vi "backup_stepper_Control.vi"   [LabVIEW 2015]
uses:
  <vilib>/eio/EIOMethodNode/EIOMethodNode.xnode
  <vilib>/rvi/eio/common/nirviEmuTemplateMethod_errors.vi
  <vilib>/eio/EIOPropertyNode/EIOPropertyNode.xnode
  <vilib>/eio/EIONode/EIONode.xnode
  Controls/Stepper SM Enumerator.ctl
  <vilib>/rvi/eio/common/nirviEmuTemplatePropertyGet_errors.vi
  <vilib>/rvi/eio/common/nirviEmuTemplatePropertyGet_noerrors.vi
  <vilib>/rvi/eio/common/nirviEmuTemplatePropertySet_errors.vi
  <vilib>/rvi/eio/common/nirviEmuTemplatePropertySet_noerrors.vi
types:
  T1 = typedef "Stepper SM Enumerator.ctl" = enum16{"Running", "Backing up", "Idle", "Home", "Lim"}
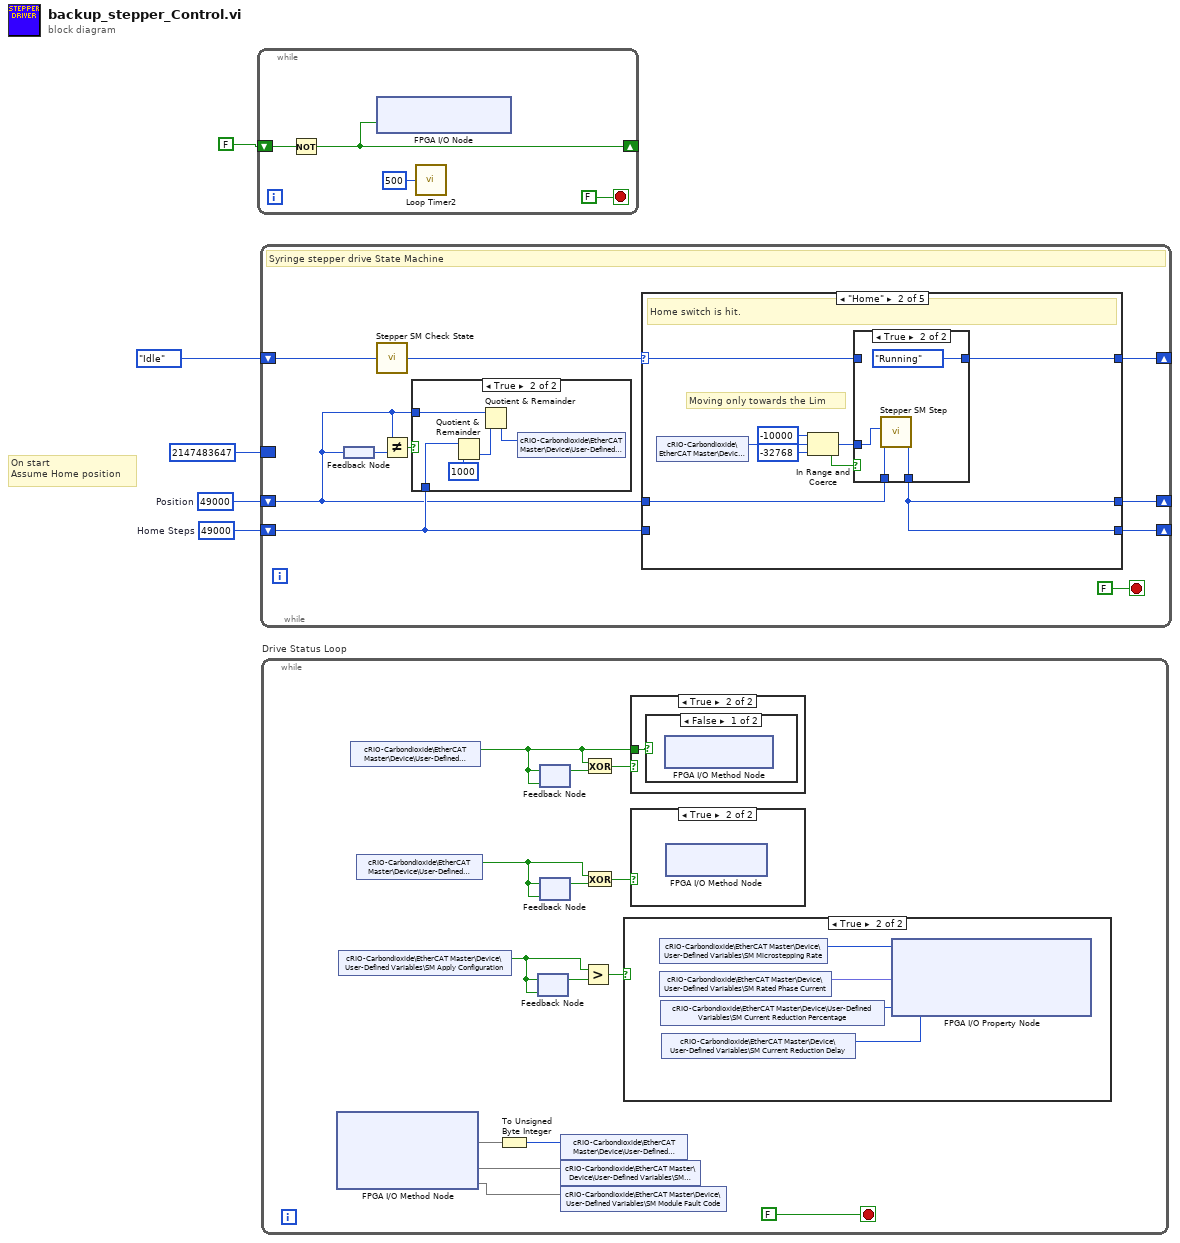
[diagram p0: block diagram]
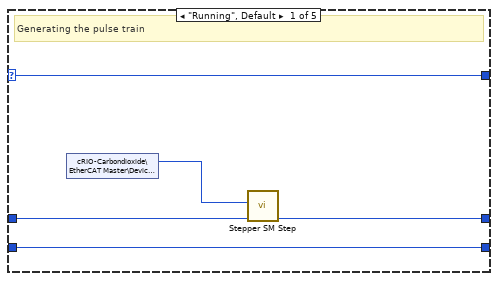
[diagram p3: hidden frame]
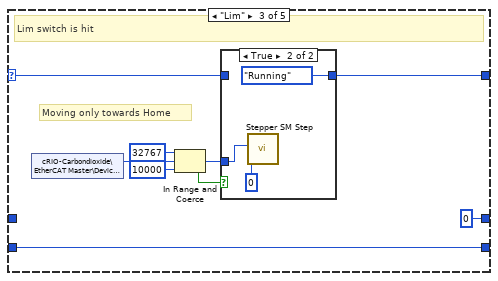
[diagram p5: hidden frame]
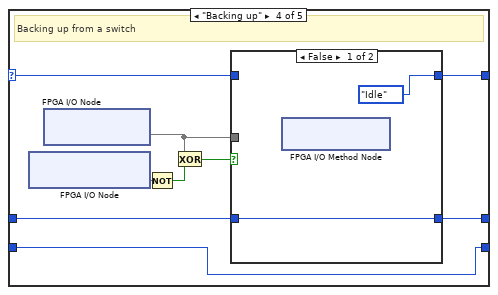
[diagram p7: hidden frame]
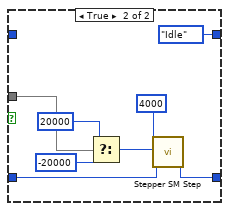
[diagram p8: hidden frame]
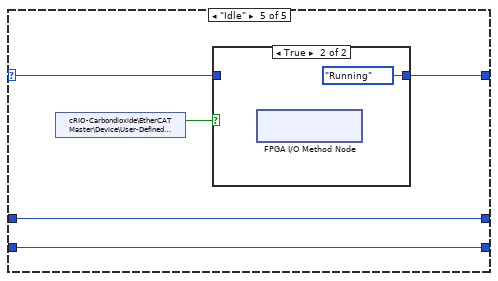
[diagram p9: hidden frame]
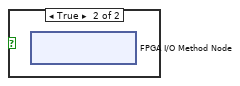
[diagram p14: hidden frame]
diagram:
  w1 = 49000  # Home Steps
  w3 = 49000  # Position
  # "On start\nAssume Home position"
  n1 = while {
    shift-right: [w7] -> _
    shift-left: FALSE ("Stepper/User LED") -> [w8]
    stop <- FALSE stop-if-true
    n2 = Not(x=w8) -> (.not. x?=w7:bool)
    n3 = xnode "FPGA I/O Node"("Stepper/User LED"=w7) -> ()  [unwired: 1 in, 1 out]
    n4 = call "Loop Timer2"("Count(mSec)"=u32 500) -> ()  [unwired: 1 out]
  }
  n5 = while {
    shift-right: [w18] -> _
    shift-left: Stepper_SM_Enumerator."Idle" -> [w17]
    shift-right: [w15] -> _
    shift-left: w3 -> [w10]
    border: 2147483647 -> [_]
    shift-right: [w13] -> _
    shift-left: w1 -> [w11]
    stop <- FALSE stop-if-true
    # "Syringe stepper drive State Machine"
    n6 = feedback-in #1(w10) -> ()
    n7 = feedback #1() -> (w12:i32)
    n8 = call "Stepper SM Check State.vi"("State in"=w17) -> ("State out"=w16:T1)
    n9 = Not Equal?(x=w10, y=w12) -> (x != y?=w14:bool)
    n10 = case shown="True" w14 {
      tunnel: w10 -> [_ w21]
      tunnel: w11 -> [_ w20]
      frame False {
      }
      frame True {
        n11 = Quotient & Remainder(x=w20, y=1000) -> (floor(x/y)=w23:i32)  [unwired: 1 out]
        n12 = Quotient & Remainder(x=w21, y=w23) -> (floor(x/y)=w22:i32)  [unwired: 1 out]
        n13 = shared-variable "cRIO-Carbondioxide\\EtherCAT Master\\Device\\User-Defined Variables\\SM Position"(w22) -> ()  [unwired: 1 in, 1 out]
      }
    }
    n14 = case shown="\"Home\"" w16 {
      selector: w16 -> [w29 w32 w48 w63 w80]
      tunnel: [w29 w33 w47 w61 w79] -> w18
      tunnel: w10 -> [w27 w31 _ w60 w78]
      tunnel: [w26 w30 0 ("Position") w59 w78] -> w15
      tunnel: [w25 w30 w46 w58 w77] -> w13
      tunnel: w11 -> [w25 _ w46 w58 w77]
      frame "Running", Default {
        # "Generating the pulse train"
        n15 = shared-variable "cRIO-Carbondioxide\\EtherCAT Master\\Device\\User-Defined Variables\\SM Ticks"() -> (w28:i16)  [unwired: 1 in, 1 out]
        n16 = call "Stepper SM Step.vi"("Step Count in"=w27, "Half period (ticks)"=w28) -> ("Step Count out"=w26:i32)  [unwired: 9 in]
      }
      frame "Home" {
        # "Moving only towards the Lim"
        # "Home switch is hit."
        n17 = shared-variable "cRIO-Carbondioxide\\EtherCAT Master\\Device\\User-Defined Variables\\SM Ticks"() -> (w38:i16)  [unwired: 1 in, 1 out]
        n18 = In Range and Coerce(upper limit=i16 -10000, x=w38, lower limit=i16 -32768) -> (coerced(x)=w37:i16, In Range?=w34:bool)
        n19 = case shown="True" w34 {
          tunnel: w37 -> [_ w43]
          tunnel: [w40 Stepper_SM_Enumerator."Running" ("State out")] -> w33
          tunnel: w32 -> [w40 _]
          tunnel: w31 -> [w39 w42]
          tunnel: [w39 w41] -> w30
          frame False {
          }
          frame True {
            n20 = call "Stepper SM Step.vi"("Step Count in"=w42, "Half period (ticks)"=w43) -> ("Step Count out"=w41:i32)  [unwired: 9 in]
          }
        }
      }
      frame "Lim" {
        # "Moving only towards Home"
        # "Lim switch is hit"
        n21 = shared-variable "cRIO-Carbondioxide\\EtherCAT Master\\Device\\User-Defined Variables\\SM Ticks"() -> (w53:i16)  [unwired: 1 in, 1 out]
        n22 = In Range and Coerce(upper limit=i16 32767, x=w53, lower limit=i16 10000) -> (coerced(x)=w52:i16, In Range?=w49:bool)
        n23 = case shown="True" w49 {
          tunnel: w52 -> [_ w56]
          tunnel: w48 -> [w54 _]
          tunnel: [w54 Stepper_SM_Enumerator."Running" ("State out")] -> w47
          frame False {
          }
          frame True {
            n24 = call "Stepper SM Step.vi"("Step Count in"=0, "Half period (ticks)"=w56) -> ()  [unwired: 9 in, 1 out]
          }
        }
      }
      frame "Backing up" {
        # "Backing up from a switch"
        n25 = xnode "FPGA I/O Node"() -> ("Stepper HOME"=w65)  [unwired: 1 in, 1 out]
        n26 = xnode "FPGA I/O Node"() -> ("Stepper LIM"=w62)  [unwired: 1 in, 1 out]
        n27 = Not(x=w65) -> (.not. x?=w64:bool)
        n28 = Exclusive Or(1:w64, 2:w62) -> (0:w66:bool)
        n29 = case shown="False" w66 {
          tunnel: w63 -> [_ _]
          tunnel: w62 -> [_ w76]
          tunnel: [Stepper_SM_Enumerator."Idle" ("State out") Stepper_SM_Enumerator."Idle" ("State out")] -> w61
          tunnel: w60 -> [w67 w70]
          tunnel: [w67 w69] -> w59
          frame False {
            n30 = xnode "FPGA I/O Method Node"() -> ()  [unwired: 1 in, 1 out]
          }
          frame True {
            n31 = Select(t=i16 20000 ("Half period (ticks)"), s=w76, f=i16 -20000 ("Half period (ticks)")) -> (s? t:f=w71:i16)
            n32 = call "Stepper SM Step.vi"("Step Count in"=w70, "Half period (ticks)"=w71, "Edges (2)"=4000) -> ("Step Count out"=w69:i32)  [unwired: 8 in]
          }
        }
      }
      frame "Idle" {
        n33 = shared-variable "cRIO-Carbondioxide\\EtherCAT Master\\Device\\User-Defined Variables\\SM Enable Drive"() -> (w81:bool)  [unwired: 1 in, 1 out]
        n34 = case shown="True" w81 {
          tunnel: w80 -> [w82 _]
          tunnel: [w82 Stepper_SM_Enumerator."Running" ("State out")] -> w79
          frame False {
          }
          frame True {
            n35 = xnode "FPGA I/O Method Node"() -> ()  [unwired: 1 in, 1 out]
          }
        }
      }
    }
  }
  n36 = while "Drive Status Loop" {
    stop <- FALSE ("stop") stop-if-true
    n37 = xnode "FPGA I/O Method Node"() -> ("Drive Status"=w87, "Module Fault?"=w86, "Module Fault Code"=w85)  [unwired: 1 in, 1 out]
    n38 = shared-variable "cRIO-Carbondioxide\\EtherCAT Master\\Device\\User-Defined Variables\\SM Apply Configuration"() -> (w88:bool)  [unwired: 1 in, 1 out]
    n39 = shared-variable "cRIO-Carbondioxide\\EtherCAT Master\\Device\\User-Defined Variables\\SM Enable Drive"() -> (w90:bool)  [unwired: 1 in, 1 out]
    n40 = shared-variable "cRIO-Carbondioxide\\EtherCAT Master\\Device\\User-Defined Variables\\SM Clear Faults"() -> (w89:bool)  [unwired: 1 in, 1 out]
    n41 = To Unsigned Byte Integer(number=w87) -> (unsigned 8bit integer=w84:u8)
    n42 = feedback-in #2(w88) -> ()
    n43 = feedback #2(w88) -> (w92:bool)
    n44 = feedback-in #3(w90) -> ()
    n45 = feedback #3(w90) -> (w95:bool)
    n46 = feedback-in #4(w89) -> ()
    n47 = feedback #4(w89) -> (w94:bool)
    n48 = shared-variable "cRIO-Carbondioxide\\EtherCAT Master\\Device\\User-Defined Variables\\SM Drive Status"(w84) -> ()  [unwired: 1 in, 1 out]
    n49 = shared-variable "cRIO-Carbondioxide\\EtherCAT Master\\Device\\User-Defined Variables\\SM Module Fault?"(w86) -> ()  [unwired: 1 in, 1 out]
    n50 = shared-variable "cRIO-Carbondioxide\\EtherCAT Master\\Device\\User-Defined Variables\\SM Module Fault Code"(w85) -> ()  [unwired: 1 in, 1 out]
    n51 = Greater?(x=w88, y=w92) -> (0:w91:bool)
    n52 = Exclusive Or(1:w95, 2:w90) -> (0:w96:bool)
    n53 = Exclusive Or(1:w94, 2:w89) -> (0:w93:bool)
    n54 = case shown="True" w91 {
      frame False {
      }
      frame True {
        n55 = shared-variable "cRIO-Carbondioxide\\EtherCAT Master\\Device\\User-Defined Variables\\SM Microstepping Rate"() -> (w101:u8)  [unwired: 1 in, 1 out]
        n56 = shared-variable "cRIO-Carbondioxide\\EtherCAT Master\\Device\\User-Defined Variables\\SM Rated Phase Current"() -> (w100:fxp<+/-,12,4>)  [unwired: 1 in, 1 out]
        n57 = shared-variable "cRIO-Carbondioxide\\EtherCAT Master\\Device\\User-Defined Variables\\SM Current Reduction Percentage"() -> (w99:u8)  [unwired: 1 in, 1 out]
        n58 = shared-variable "cRIO-Carbondioxide\\EtherCAT Master\\Device\\User-Defined Variables\\SM Current Reduction Delay"() -> (w98:u16)  [unwired: 1 in, 1 out]
        n59 = xnode "FPGA I/O Property Node"("Microstepping Rate"=w101, "Rated Phase Current"=w100, "Current Reduction Percentage"=w99, "Current Reduction Delay"=w98) -> ()  [unwired: 1 in, 1 out]
      }
    }
    n60 = case shown="True" w96 {
      tunnel: w90 -> [_ w102]
      frame False {
      }
      frame True {
        n61 = case shown="False" w102 {
          frame False {
            n62 = xnode "FPGA I/O Method Node"() -> ()  [unwired: 1 in, 1 out]
          }
          frame True {
            n63 = xnode "FPGA I/O Method Node"() -> ()  [unwired: 1 in, 1 out]
          }
        }
      }
    }
    n64 = case shown="True" w93 {
      frame False {
      }
      frame True {
        n65 = xnode "FPGA I/O Method Node"() -> ()  [unwired: 1 in, 1 out]
      }
    }
  }
